vi "GetEvtReports.vi"(8 "error in (no error)":errorcluster, 11 "EventPluginBaseClass in":refnum<class "EventPluginBaseClass.lvclass">) -> (0 "error out":errorcluster, 3 "EventPluginBaseClass out":refnum<class "EventPluginBaseClass.lvclass">)   [LabVIEW 2017, in "EventPlugins.lvlib" / "EventPluginBaseClass.lvclass"]
uses:
  EventPluginBaseClass.lvclass
  <userlib>/NIST/BaseClasses/Object_class/BaseObject.lvclass
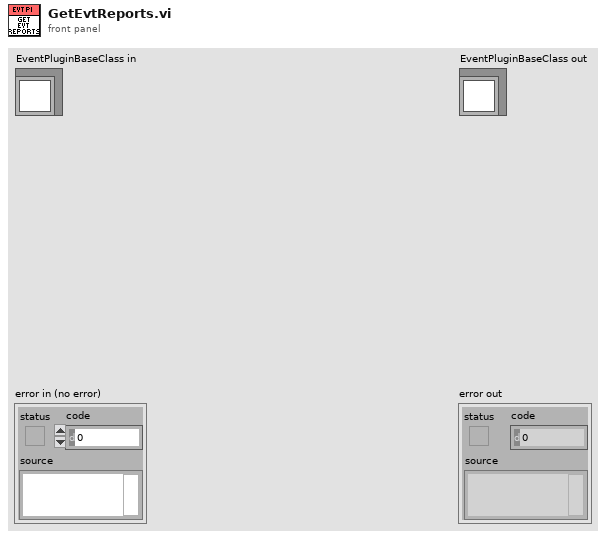
[diagram p1: front panel]
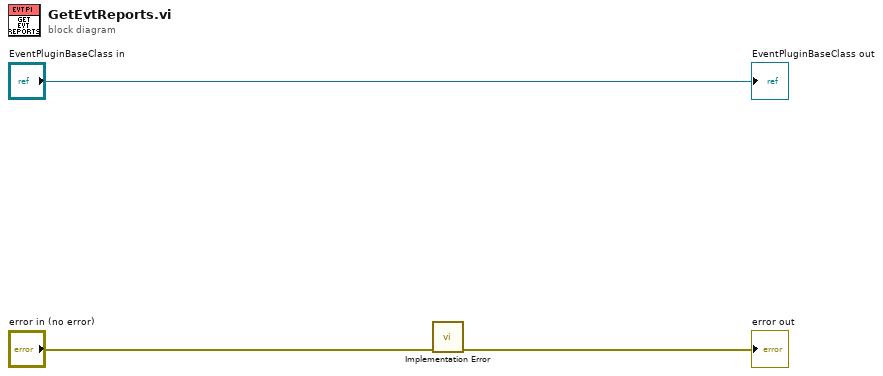
[diagram p0: block diagram]
diagram:
  n1 = call <userlib>:"Implementation Error.vi"("error in (no error)"="error in (no error)") -> ("error out"=→"error out":errorcluster)  [unwired: 10 in]
  "EventPluginBaseClass out" <- "EventPluginBaseClass in"
